vi "save data.vi"(10 "Sample\nconcentrations":dbl[](array[numeric]) format="%.2e", 11 "file path":refnum<file>) -> ()   [LabVIEW 2015]
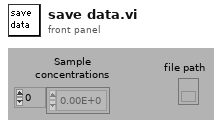
[diagram p1: front panel]
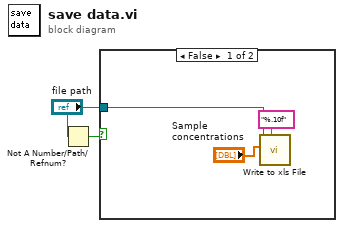
[diagram p0: block diagram]
diagram:
  n1 = Not A Number/Path/Refnum?(number/path/refnum="file path") -> (NaN/Path/Refnum?=w1:bool)
  n2 = case shown="False" w1 {
    tunnel: "file path" -> [w4 _]
    frame False {
      n3 = call "Write to xls File.vi"("format (%.3f)"="%.10f", "1D data"="Sample\nconcentrations", "refnum"=w4) -> ()  [unwired: 7 in, 2 out]
    }
    frame True {
    }
  }
